vi "generic hardware init.vi"(11 "Template in":refnum<class "Template.lvclass">) -> (0 "error out":errorcluster, 3 "Template out":refnum<class "Template.lvclass">)   [LabVIEW 2020, in "Template.lvlib" / "Template.lvclass"]
doc: "Executes any hardware initialization procedure here. Bundle the references and start-up data in the actor's private data.\nUse the parent's APIs to call the ActorConfiguiation cluster as exemplified in the parent method\nThis vi is called in the Pre Launch Init override of the Actor Framework overrides."
uses:
  Template.lvclass
  Template.lvclass/Template.ctl
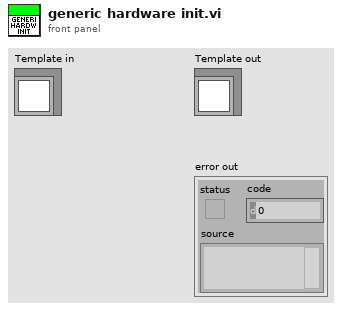
[diagram p1: front panel]
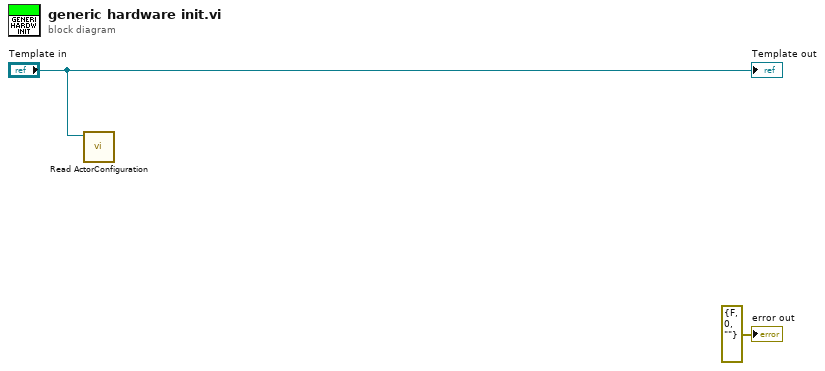
[diagram p0: block diagram]
diagram:
  n1 = call "Read ActorConfiguration.vi"("Template in"="Template in") -> ()  [unwired: 10 in, 1 out]
  "error out" <- errorcluster {"status"=FALSE, "code"=0, "source"=""} ("error out")
  "Template out" <- "Template in"
